vi "log_message.vi"(6 "timestamp":timestamp, 7 "context":string, 8 "error in (no error)":errorcluster, 9 "level":T1=400 items=["OFF"=0, "FATAL"=100, "ERROR"=200, "WARN"=300, "INFO"=400, "DEBUG"=500, "TRACE"=600, "ALL"=65535], 10 "message":string, 11 "Queue Log Provider in":refnum<class "NIErrLog Log Provider.lvclass">) -> (0 "error out":errorcluster, 3 "Queue Log Provider out":refnum<class "NIErrLog Log Provider.lvclass">)   [LabVIEW 2019, in "LVCOOOP.lvlib" / "Support API.lvlib" / "NIErrLog Log Provider.lvclass"]
uses:
  NIErrLog Log Provider.lvclass
  Log Service/public/level.ctl
  Log Service/Log Service.lvclass
  <vilib>/Utility/SystemLogging/NI_SystemLogging.lvlib
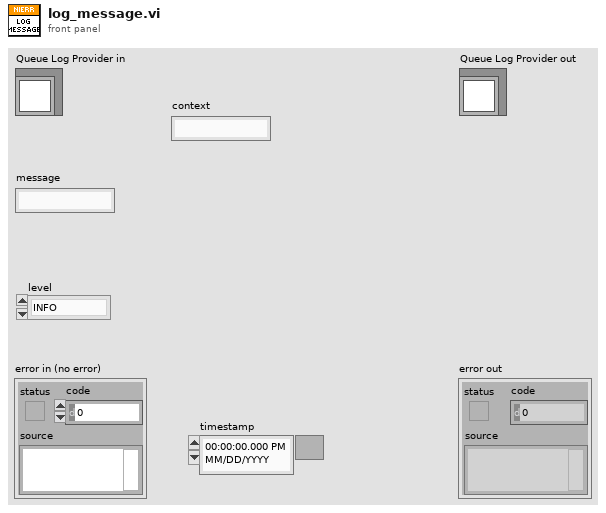
[diagram p1: front panel]
types:
  T1 = typedef "LVCOOOP.lvlib/Support API.lvlib/Log Service.lvclass/level.ctl" = u16
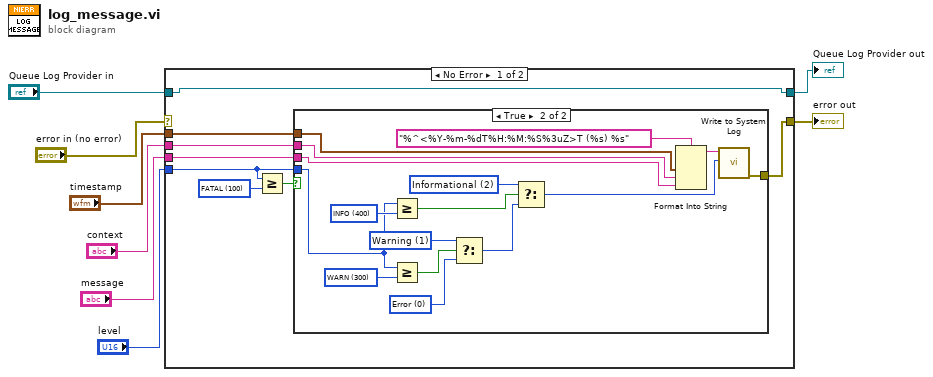
[diagram p0: block diagram]
diagram:
  n1 = case shown="No Error" "error in (no error)" {
    selector: "error in (no error)" -> [_ w34]
    tunnel: [w13 w34] -> w8
    tunnel: "timestamp" -> [w9 _]
    tunnel: "level" -> [w14 _]
    tunnel: "context" -> [w11 _]
    tunnel: "message" -> [w10 _]
    tunnel: [w16 w33] -> w2
    tunnel: "Queue Log Provider in" -> [w16 w33]
    frame No Error {
      w15 = T1 100 items=["OFF"=0, "FATAL"=100, "ERROR"=200, "WARN"=300, "INFO"=400, "DEBUG"=500, "TRACE"=600, "ALL"=65535] ("level")
      n2 = Greater Or Equal?(x=w14, y=w15) -> (x >= y?=w12:bool)
      n3 = case shown="True" w12 {
        tunnel: w14 -> [_ w25]
        tunnel: [_ w22] -> w13
        tunnel: w11 -> [_ w18]
        tunnel: w10 -> [_ w17]
        tunnel: w9 -> [_ w19]
        frame False {
        }
        frame True {
          w24 = 0 items=["Error", "Warning", "Informational"] ("severity")
          w27 = 1 items=["Error", "Warning", "Informational"] ("severity")
          w29 = T1 300 items=["OFF"=0, "FATAL"=100, "ERROR"=200, "WARN"=300, "INFO"=400, "DEBUG"=500, "TRACE"=600, "ALL"=65535] ("level")
          w30 = 2 items=["Error", "Warning", "Informational"] ("severity")
          w32 = T1 400 items=["OFF"=0, "FATAL"=100, "ERROR"=200, "WARN"=300, "INFO"=400, "DEBUG"=500, "TRACE"=600, "ALL"=65535] ("level")
          n4 = Greater Or Equal?(x=w25, y=w32) -> (x >= y?=w31:bool)
          n5 = Greater Or Equal?(x=w25, y=w29) -> (x >= y?=w28:bool)
          n6 = Select(t=w27, s=w28, f=w24) -> (s? t:f=w26:i32)
          n7 = Select(t=w30, s=w31, f=w26) -> (s? t:f=w23:i32)
          n8 = Format Into String(format string="%^<%Y-%m-%dT%H:%M:%S%3uZ>T (%s) %s", w19, w18, w17) -> (resulting string=w20:string)  [unwired: 2 in, 1 out]
          n9 = call <vilib>:"Write to System Log.vi"("severity"=w23, "message"=w20) -> ("error out"=w22:errorcluster)  [unwired: 9 in]
        }
      }
    }
    frame Error {
    }
  }
  "error out" <- w8
  "Queue Log Provider out" <- w2
